vi "Complete 1 Round - Unique Movement Order.vi"(1 "Elves in":T2(c390)) -> (0 "Elves out":T2(c390))   [LabVIEW 2020, in "AoC 2022.lvlib"]
uses:
  AoC 2022.lvlib
  Day 15 - Beacon Exclusion Zone/private/Location.ctl
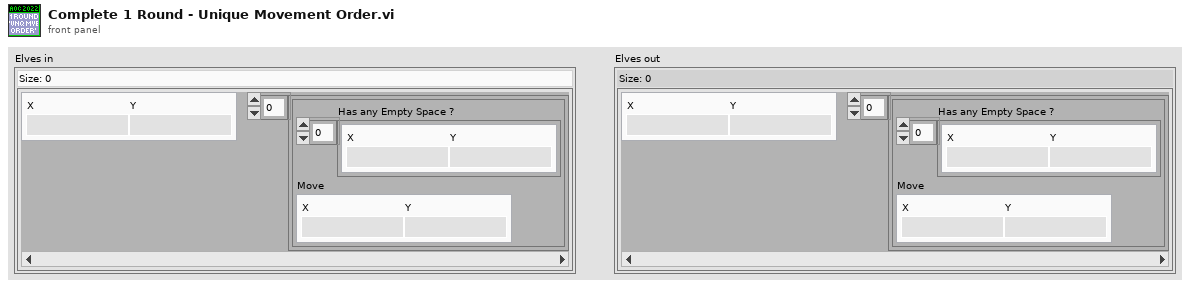
[diagram p1: front panel]
types:
  T1 = typedef "AoC 2022.lvlib/Location.ctl" = cluster{"X":i32, "Y":i32}
  T2 = map{T1, cluster{"Has any Empty Space ?":T1[], "Move":T1}[]}
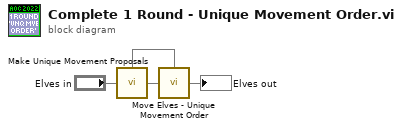
[diagram p0: block diagram]
diagram:
  n1 = call "Make Unique Movement Proposals.vi"("Elves in"="Elves in") -> ("Elves' Movement Proposals"=w2:map{T1, T1}, "Elves out"=w1:T2)
  n2 = call "Move Elves - Unique Movement Order.vi"("Elves in"=w1, "Elves' Movement Proposals"=w2) -> ("Elves out"=→"Elves out":T2)
